vi "Scan.vi"(6 "Function":i32, 8 "error in (no error)":errorcluster caption="entrée d'erreur (pas d'erreur)", 9 "Single":bool, 10 "Index":i32 caption="Index du Point" min=-15 max=15 step=1, 11 "ExperimentIn":refnum<class "Experiment.lvclass"> caption="DNL_LabVIEW Object in") -> (0 "error out":errorcluster caption="sortie d'erreur", 1 "TimesArray":u32[](array[numeric]), 2 "ScanParsOut":dbl[](array[numeric]), 3 "ExperimentOut":refnum<class "Experiment.lvclass"> caption="DNL_LabVIEW Object out")   [LabVIEW 2019, in "Experiment.lvclass"]
uses:
  Experiment.lvclass
  Experiment.lvclass/Experiment.ctl
  DevicesClass/BaseDevice/BaseDevice.lvclass
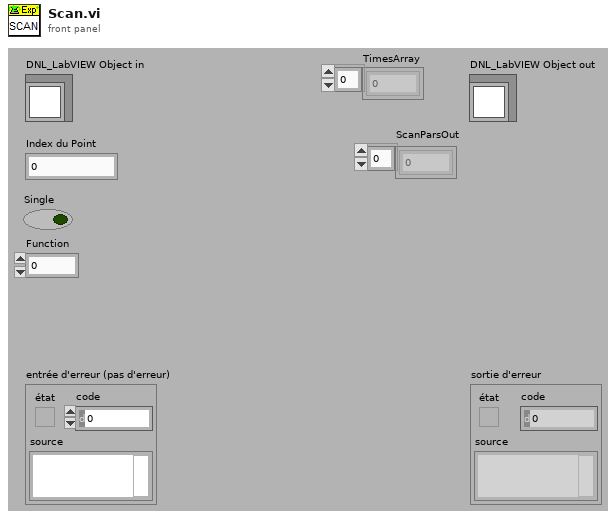
[diagram p1: front panel]
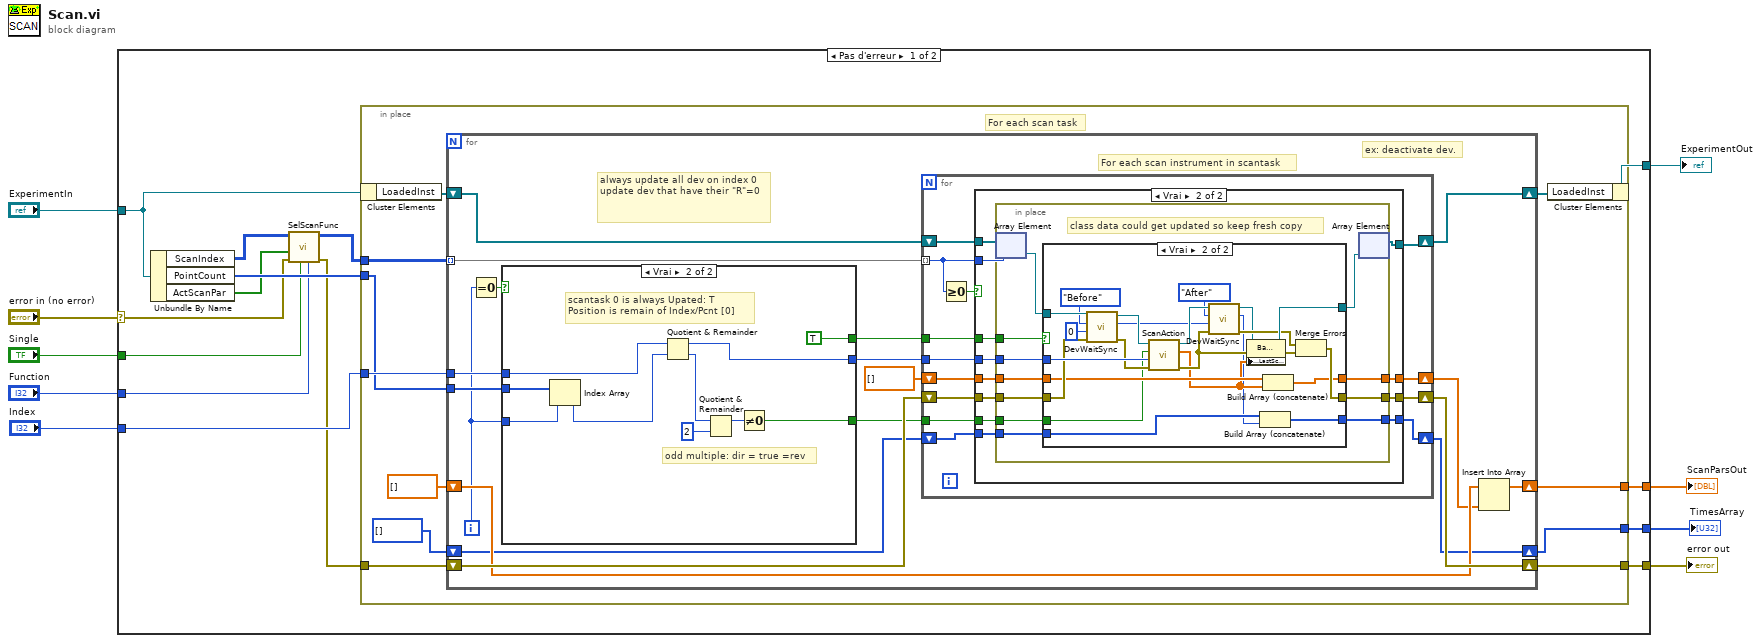
[diagram p0: block diagram]
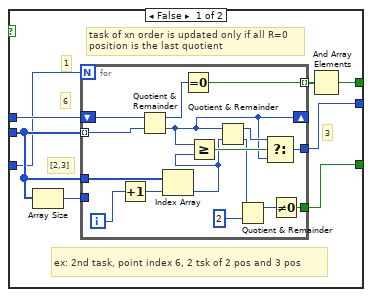
[diagram p2: hidden frame]
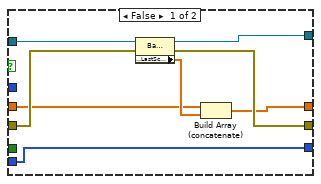
[diagram p4: hidden frame]
diagram:
  n1 = case shown="Pas d'erreur" "error in (no error)" {
    selector: "error in (no error)" -> [w13 w159]
    tunnel: [w22 w159] -> w8
    tunnel: [w20 w158] -> w6
    tunnel: "ExperimentIn" -> [w19 w158]
    tunnel: "Index" -> [w23 _]
    tunnel: [w21 _] -> w4
    tunnel: "Function" -> [w10 _]
    tunnel: "Single" -> [w11 _]
    tunnel: [w17 _] -> w1
    frame No Error {
      n2 = Unbundle By Name(w19) -> ("ScanIndex"=w15:i32[][], "PointCount"=w18:i32[], "ActScanPar"=w14:bool[])
      n3 = call "SelScanFunc.vi"("Function"=w10, "SInglePar"=w11, "ErrorIn(No Error)"=w13, "Active ScanPar"=w14, "ScanIndexIn"=w15) -> ("sortie d'erreur"=w12:errorcluster, "ScanIndexOut"=w16:i32[][])  [unwired: 4 in, 1 out]
      n4 = in-place {
        in-place-border: w23 -> [w34]
        in-place-border: [w33] -> w22
        in-place-border: w12 -> [w32]
        in-place-border: [w30] -> w21
        in-place-border: w16 -> [w27]
        in-place-border: w18 -> [w26]
        in-place-border: [w24] -> w17
        # "For each scan task"
        n5 = in-place-cluster #1(w19) -> ("LoadedInst"=w29:refnum<class "BaseDevice.lvclass">[])
        n6 = for {
          tunnel: w27 -> [w52] mode=indexing
          shift-right: [w46] -> w28
          shift-left: w29 -> [w51]
          tunnel: w26 -> [w43]
          tunnel: w34 -> [w50]
          shift-right: [w48] -> w33
          shift-left: w32 -> [w47]
          shift-right: [w44] -> w30
          shift-left: dbl[] [] -> [w45]
          shift-right: [w35] -> w24
          shift-left: u32[] [] -> [w36]
          i -> [w40]
          # "For each scan instrument in scantask"
          # "always update all dev on index 0\nupdate dev that have their \"R\"=0"
          # "ex: deactivate dev."
          n7 = Equal To 0?(x=w40) -> (x = 0?=w42:bool)
          n8 = case shown="Vrai" w42 {
            tunnel: [w60 TRUE] -> w41
            tunnel: w50 -> [w59 w82]
            tunnel: [w55 w81] -> w49
            tunnel: w43 -> [w57 w84]
            tunnel: w40 -> [w54 w85]
            tunnel: [w53 w77] -> w37
            frame False {
              # "3"
              # "1"
              # "ex: 2nd task, point index 6, 2 tsk of 2 pos and 3 pos"
              # "6"
              # "[2,3]"
              # "task of xn order is updated only if all R=0\nposition is the last quotient"
              n9 = Array Size(array=w57) -> (size(s)=w56:i32)
              n10 = for {
                N: w54 -> [_]
                shift-right: [w67] -> _
                shift-left: w59 -> [w74]
                tunnel: w57 -> [w72] mode=indexing
                tunnel: [w75] -> w58 mode=indexing
                tunnel: w57 -> [w73]
                tunnel: w56 -> [_]
                tunnel: [w66] -> w55
                tunnel: [w62] -> w53
                i -> [w71]
                n11 = Increment(x=w71) -> (x+1=w70:i32)
                n12 = Quotient & Remainder(x=w74, y=w72) -> (x-y*floor(x/y)=w76:i32, floor(x/y)=w67:i32)
                n13 = Index Array(array=w73, index=w70) -> (element=w61:i32)
                n14 = Equal To 0?(x=w76) -> (x = 0?=w75:bool)
                n15 = Greater Or Equal?(x=w67, y=w61) -> (x >= y?=w68:bool)
                n16 = Quotient & Remainder(x=w67, y=w61) -> (x-y*floor(x/y)=w69:i32, floor(x/y)=w63:i32)
                n17 = Quotient & Remainder(x=w63, y=2) -> (x-y*floor(x/y)=w65:i32)  [unwired: 1 out]
                n18 = Select(t=w69, s=w68, f=w67) -> (s? t:f=w66:i32)
                n19 = Not Equal To 0?(x=w65) -> (x != 0?=w62:bool)
              }
              n20 = And Array Elements(Boolean array=w58) -> (logical AND=w60:bool)
            }
            frame True {
              # "odd multiple: dir = true =rev"
              # "scantask 0 is always Upated: T\nPosition is remain of Index/Pcnt [0]"
              n21 = Index Array(array=w84, index=w85) -> (element=w83:i32)
              n22 = Quotient & Remainder(x=w82, y=w83) -> (x-y*floor(x/y)=w81:i32, floor(x/y)=w80:i32)
              n23 = Quotient & Remainder(x=w80, y=2) -> (x-y*floor(x/y)=w78:i32)  [unwired: 1 out]
              n24 = Not Equal To 0?(x=w78) -> (x != 0?=w77:bool)
            }
          }
          n25 = for {
            tunnel: w52 -> [w87] mode=indexing
            tunnel: w41 -> [w99]
            tunnel: w49 -> [w98]
            shift-right: [w97] -> w48
            shift-left: w47 -> [w96]
            shift-right: [w94] -> w46
            shift-left: w51 -> [w95]
            shift-right: [w93] -> w38
            shift-left: dbl[] [] -> [w92]
            tunnel: w37 -> [w91]
            shift-right: [w90] -> w35
            shift-left: w36 -> [w89]
            n26 = Greater Or Equal To 0?(x=w87) -> (x >= 0?=w88:bool)
            n27 = case shown="Vrai" w88 {
              tunnel: w99 -> [_ w115]
              tunnel: w98 -> [_ w114]
              tunnel: [w101 w113] -> w97
              tunnel: w96 -> [w101 w112]
              tunnel: w95 -> [w103 w111]
              tunnel: [w103 w110] -> w94
              tunnel: w87 -> [_ w109]
              tunnel: [w102 w108] -> w93
              tunnel: w92 -> [w102 w107]
              tunnel: w91 -> [_ w106]
              tunnel: [w100 w105] -> w90
              tunnel: w89 -> [w100 w104]
              frame False {
                # "Empty ScanArr line Ends =-1"
              }
              frame True {
                n28 = in-place {
                  in-place-border: w115 -> [w126]
                  in-place-border: w114 -> [w125]
                  in-place-border: [w124] -> w113
                  in-place-border: w112 -> [w123]
                  in-place-border: [w120] -> w108
                  in-place-border: w107 -> [w119]
                  in-place-border: w106 -> [w118]
                  in-place-border: [w117] -> w105
                  in-place-border: w104 -> [w116]
                  # "class data could get updated so keep fresh copy"
                  n29 = in-place-array #2(w111, w109) -> (w122:refnum<class "BaseDevice.lvclass">)
                  n30 = case shown="Vrai" w126 {
                    tunnel: w122 -> [w134 w153]
                    tunnel: [w133 w155] -> w121
                    tunnel: w125 -> [_ w157]
                    tunnel: w123 -> [w132 w154]
                    tunnel: [w131 w148] -> w124
                    tunnel: [w129 w144] -> w120
                    tunnel: w119 -> [w128 w143]
                    tunnel: w118 -> [_ w138]
                    tunnel: [w127 w137] -> w117
                    tunnel: w116 -> [w127 w136]
                    frame False {
                      n31 = property class="BaseDevice.lvclass"(reference=w134, error in=w132) -> (reference out=w133:refnum<class "BaseDevice.lvclass">, error out=w131:errorcluster, "Accessor:LastScanPos"=w130:dbl[])
                      n32 = Build Array (concatenate)(w128, w130) -> (w129:dbl[])
                    }
                    frame True {
                      n33 = call "DevWaitSync.vi"("error in (no error)"=w154, "Time in"=u32 0, "Type"=enum16{"After", "Before"}."Before", "BaseDevice en entrée"=w153) -> ("error out"=w151:errorcluster, "Time"=w141:u32, "BaseDevice en sortie"=w152:refnum<class "BaseDevice.lvclass">)  [unwired: 5 in]
                      n34 = call-dynamic "ScanAction.vi"("error in (no error)"=w151, "IndicePoint"=w157, "Dir"=w138, "Device en entrée"=w152) -> ("error out"=w149:errorcluster, "ScanParsOut"=w139:dbl[], "Device en sortie"=w150:refnum<class "BaseDevice.lvclass">)  [unwired: 5 in]
                      n35 = call "DevWaitSync.vi"("error in (no error)"=w149, "Time in"=w141, "Type"=enum16{"After", "Before"}."After", "BaseDevice en entrée"=w150) -> ("error out"=w147:errorcluster, "Time"=w135:u32, "BaseDevice en sortie"=w140:refnum<class "BaseDevice.lvclass">)  [unwired: 5 in]
                      n36 = property class="BaseDevice.lvclass"(reference=w140, error in=w149, "Accessor:LastScanPos"=w139) -> (reference out=w155:refnum<class "BaseDevice.lvclass">, error out=w156:errorcluster)
                      n37 = Build Array (concatenate)(w136, w135) -> (w137:u32[])
                      n38 = Build Array (concatenate)(w143, w139) -> (w144:dbl[])
                      n39 = Merge Errors(w147, w156) -> (w148:errorcluster)
                    }
                  }
                  n40 = in-place-array #2(w121) -> (w110:refnum<class "BaseDevice.lvclass">[])  [unwired: 1 out]
                }
              }
            }
          }
          n41 = Insert Into Array(array=w45, new element=w38) -> (w44:dbl[])  [unwired: 1 in]
        }
        n42 = in-place-cluster #1("LoadedInst"=w28) -> (w20:refnum<class "Experiment.lvclass">)
      }
    }
    frame Error {
    }
  }
  "error out" <- w8
  "ExperimentOut" <- w6
  "ScanParsOut" <- w4
  "TimesArray" <- w1
